vi "DAQmx.44xx.Get DAQ Type from Device.vi"(8 "error in (no error)":errorcluster, 11 "DAQmx Device Name":tag) -> (0 "error out":errorcluster, 2 "DAQ Type":T1, 3 "DevIsSimulated":bool)   [LabVIEW 2019, in "DAQmx.lvclass"]
uses:
  DAQmx.lvclass
  typedefs/DAQ.Config.Device Type--enum.ctl
  <resource>/objmgr/daqmx.rc
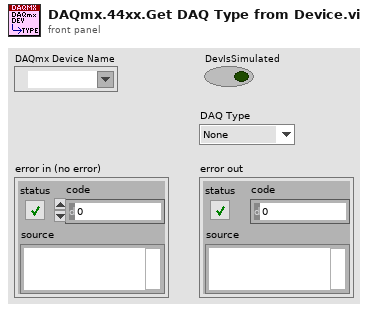
[diagram p1: front panel]
types:
  T1 = typedef "DAQmx.lvclass/DAQ.Config.Device Type--enum.ctl" = enum16{"None", "USB-4431", "PXI-446x"}
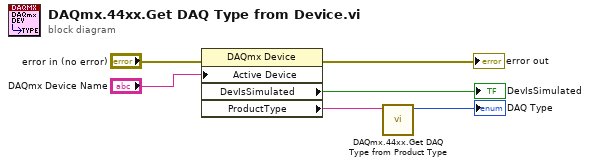
[diagram p0: block diagram]
diagram:
  n1 = property class="DAQmx Device"(error in="error in (no error)", "Active Device"="DAQmx Device Name") -> (error out=→"error out":errorcluster, "DevIsSimulated"=→"DevIsSimulated":bool, "ProductType"=w6:string)  [unwired: 1 in, 1 out]
  n2 = call "DAQmx.44xx.Get DAQ Type from Product Type.vi"("ProductType"=w6) -> ("DAQ Type"=→"DAQ Type":T1)  [unwired: 10 in]
